vi "GF_AgilentQuery.vi"(7 "error in (no error)":errorcluster, 8 "Timeout":u32, 9 "Query":string, 10 "Session In":refnum<visa-resource-name>) -> (0 "error out":errorcluster, 2 "Token Array 2":cluster{"Name":string, "Value":string}[](array[cluster]), 3 "Session out":refnum<visa-resource-name>)   [LabVIEW 2020]
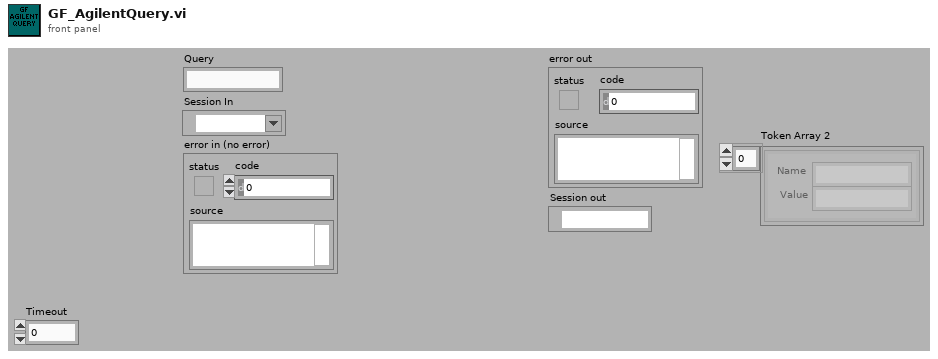
[diagram p1: front panel]
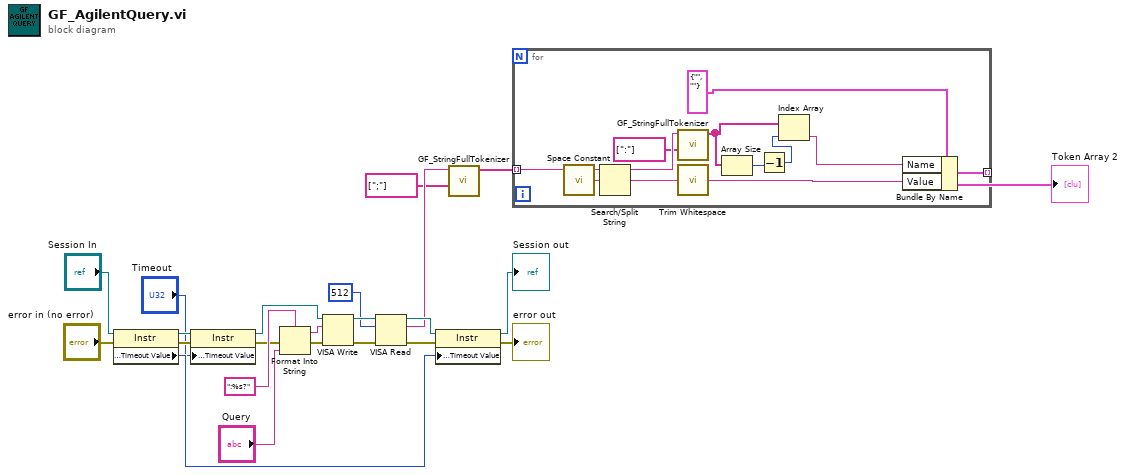
[diagram p0: block diagram]
diagram:
  n1 = property on="Property Node" class="Instr"(reference="Session In", error in="error in (no error)") -> (reference out=w20:refnum<visa-resource-name>, error out=w19:errorcluster, "General Settings:Timeout Value"=w17:u32)
  n2 = property on="Property Node" class="Instr"(reference=w20, error in=w19, "General Settings:Timeout Value"="Timeout") -> (reference out=w18:refnum<visa-resource-name>, error out=w4:errorcluster)
  n3 = Format Into String(format string=":%s?", error in=w4, "Query") -> (resulting string=w23:string, error out=w3:errorcluster)  [unwired: 1 in]
  n4 = VISA Write(VISA resource name=w18, write buffer=w23, error in (no error)=w3) -> (VISA resource name out=w21:refnum<visa-resource-name>, error out=w22:errorcluster)  [unwired: 1 out]
  n5 = VISA Read(VISA resource name=w21, byte count=u32 512, error in (no error)=w22) -> (VISA resource name out=w14:refnum<visa-resource-name>, read buffer=w8:string, error out=w15:errorcluster)  [unwired: 1 out]
  n6 = property on="Property Node" class="Instr"(reference=w14, error in=w15, "General Settings:Timeout Value"=w17) -> (reference out=→"Session out":refnum<visa-resource-name>, error out=→"error out":errorcluster)
  n7 = call "GF_StringFullTokenizer.vi"("delimiters (\\s,\\t,\\r,\\n)"=string[] [";"] ("delimiters (\\s,\\t,\\r,\\n)"), "Input String"=w8) -> ("Token Array"=w6:string[])  [unwired: 9 in]
  n8 = for {
    tunnel: w6 -> [w35] mode=indexing
    tunnel: [w32] -> w2 mode=indexing
    n9 = call <vilib>:"Space Constant.vi"() -> ("String"=w34:string)
    n10 = Search/Split String(string=w35, search string/char (-)=w34) -> (substring before match=w29:string, match + rest of string=w30:string)  [unwired: 1 in, 1 out]
    n11 = call "GF_StringFullTokenizer.vi"("delimiters (\\s,\\t,\\r,\\n)"=string[] [":"] ("delimiters (\\s,\\t,\\r,\\n)"), "Input String"=w29) -> ("Token Array"=w25:string[])  [unwired: 9 in]
    n12 = call <vilib>:"Trim Whitespace.vi"("string"=w30) -> ("trimmed string"=w31:string)  [unwired: 1 in]
    n13 = Array Size(array=w25) -> (size(s)=w27:i32)
    n14 = Decrement(x=w27) -> (x-1=w26:i32)
    n15 = Index Array(array=w25, index=w26) -> (element=w24:string)
    n16 = Bundle By Name(cluster=cluster{"Name":string, "Value":string} {"Name"="", "Value"=""} ("Cluster"), "Name"=w24, "Value"=w31) -> (w32:cluster{"Name":string, "Value":string})
  }
  "Token Array 2" <- w2
